vi "Pressure Control 1.vi"() -> ()   [LabVIEW 2013]
uses:
  <vilib>/DAQmx/write.llb/DAQmx Write.vi
  <vilib>/DAQmx/write.llb/DAQmx Write (Digital Bool 1Line 1Point).vi
  <vilib>/DAQmx/read.llb/DAQmx Read.vi
  <vilib>/DAQmx/read.llb/DAQmx Read (Analog DBL 1Chan 1Samp).vi
  <vilib>/Analysis/1siggen.llb/Ramp Pattern by Samples.vi
  support files/Pr Data Global.vi
  <vilib>/DAQmx/miscellaneous.llb/DAQmx Fill In Error Info.vi
  <vilib>/Analysis/NI_AALPro.lvlib
  <vilib>/Analysis/NI_AALBase.lvlib
panel:
  out "Delay Start":dbl format="%.2f"
  in  "Start Test":bool
  in  "quit":bool
  out "loops":bool
  out "Running?":bool
  in  "Tab":T1(tab)
  out "Vac":bool
  out "File Data:":T2 {"Min." format="%.2f"; "Ave." format="%.2f"; "Max." format="%.2f"}
  out "units 2":string
  out "units 1":string
  out "Relief":bool
  out "Pressure":bool
  out "Pr Data":sgl(graph)
  out "Ave. Pressure Input":sgl format="%.2f"
  out "Pressure Input":sgl format="%.2f"
  out "units 4":string
  out "units 3":string
  in  "Config Cluster":T3={"Pressure Setpoint"=20.0, "Deadband"=2.0, "Data Read Rate"=10.0, "Data Location"=1, "# Points to Ave."=2, "Data Storage"=FALSE, "Data Storage Rate"=10.0, "Data Path"=path "", "TR #"="", "Comp. ID"="", "Reset Buffer"=FALSE, "Reponse Time"=2.0} {"Reponse Time" min=0.0 max=10.0 format="%.1f"; "Data Storage Rate" format="%<%H:%M:%S>t"; "# Points to Ave." min=1 max=10000; "Data Location" min=1 max=10; "Data Read Rate" min=0.1 max=3600.0 format="%.1f"; "Deadband" format="%.2f"; "Pressure Setpoint" format="%.2f"}
  in  "IO Settings":T4={"Feedback Settings"={"Comm Resource"="Pr Module", "Device"="AI 120", "Item"="Channel 0"}, "Pressure Valve"={"Comm Resource"="Pr Module", "Device"="Relay", "Item"="Channel 0"}, "Relief Valve"={"Comm Resource"="Pr Module", "Device"="Relay", "Item"="Channel 0"}, "Vacuum Valve"={"Comm Resource"="Pr Module", "Device"="Relay", "Item"="Channel 0"}}
  in  "get amps":bool[](array[boolean])=[FALSE, FALSE, FALSE, FALSE, FALSE, FALSE]
  out "XY Graph":cluster{"Ramp Pattern":dbl[], dbl[]}[](graph)
  in  "Re-Calc":bool
  in  "Pr. Cal.":T5={"Model"="", "Gage #"="", "Cal Date"="", "Eng. Units"=[0.0, 0.0, 0.0, 0.0, 0.0, 0.0], "Amps"=[0.0, 0.0, 0.0, 0.0, 0.0, 0.0], "# Cal Points"=5, "Offset"=0.0, "Slope"=0.0, "Units"="kPa", "Master Gage #"=""} {"Slope" format="%.4f"; "Offset" format="%.4f"; "# Cal Points" min=2 max=6; "Amps" format="%.3f"; "Eng. Units" format="%.3f"}
  out "Data":sgl[][](array[numeric]) format="%.2f"
  # "(0.1-3600)"
  # "(0-10)"
  # "(1-10000)"
  # "(1-10)"
  # "(hh:mm:ss)"
  # "Pressure Input"
  # "(2-6)"
  # "min."
  # "max."
  # "ave."
  # "1"
  # "2"
  # "3"
  # "4"
  # "5"
  # "6"
  # "7"
  # "8"
  # "9"
  # "10"
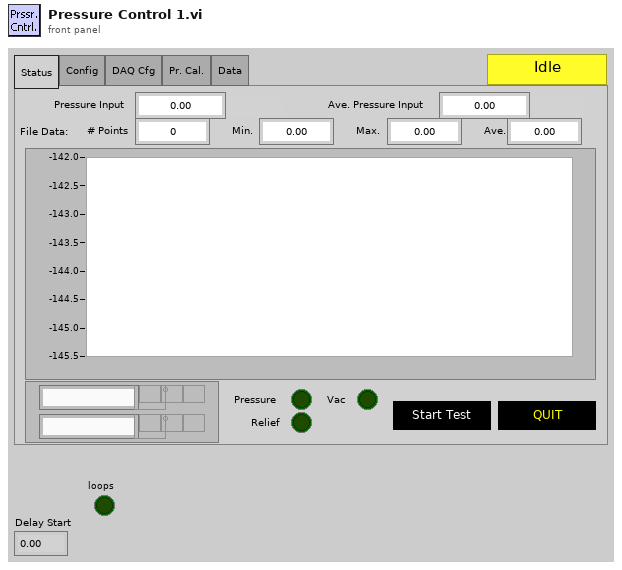
[diagram p1: front panel]
types:
  T1 = enum32{"Status", "Config", "DAQ Cfg", "Pr. Cal.", "Data"}
  T2 = cluster{"# Points":sgl, "Min.":sgl, "Max.":sgl, "Ave.":sgl}
  T3 = cluster{"Pressure Setpoint":dbl, "Deadband":dbl, "Data Read Rate":dbl, "Data Location":i32, "# Points to Ave.":i32, "Data Storage":bool, "Data Storage Rate":dbl, "Data Path":path, "TR #":string, "Comp. ID":string, "Reset Buffer":bool, "Reponse Time":dbl}
  T4 = cluster{"Feedback Settings":cluster{"Comm Resource":string, "Device":string, "Item":string}, "Pressure Valve":cluster{"Comm Resource":string, "Device":string, "Item":string}, "Relief Valve":cluster{"Comm Resource":string, "Device":string, "Item":string}, "Vacuum Valve":cluster{"Comm Resource":string, "Device":string, "Item":string}}
  T5 = cluster{"Model":string, "Gage #":string, "Cal Date":string, "Eng. Units":sgl[], "Amps":sgl[], "# Cal Points":u32, "Offset":sgl, "Slope":sgl, "Units":string, "Master Gage #":string}
  T6 = enum16{"Idle", "Adding Pr.", "Relieving Pr.", "Response Delay"}
  T7 = cluster{"IO Settings":cluster{"Feedback Settings":cluster{"Comm Resource":string, "Device":string, "Item":string}, "Pressure Valve":cluster{"Comm Resource":string, "Device":string, "Item":string}, "Relief Valve":cluster{"Comm Resource":string, "Device":string, "Item":string}, "Vacuum Valve":cluster{"Comm Resource":string, "Device":string, "Item":string}}, "Config Cluster":cluster{"Pressure Setpoint":dbl, "Deadband":dbl, "Data Read Rate":dbl, "Data Location":i32, "# Points to Ave.":i32, "Data Storage":bool, "Data Storage Rate":dbl, "Data Path":path, "TR #":string, "Comp. ID":string, "Reset Buffer":bool, "Reponse Time":dbl}, "Pr. Cal.":cluster{"Model":string, "Gage #":string, "Cal Date":string, "Eng. Units":sgl[], "Amps":sgl[], "# Cal Points":u32, "Offset":sgl, "Slope":sgl, "Units":string, "Master Gage #":string}}
  T8 = cluster{"# Pts, Min, Max, Ave.[0]":sgl, "# Pts, Min, Max, Ave.[1]":sgl, "# Pts, Min, Max, Ave.[2]":sgl, "# Pts, Min, Max, Ave.[3]":sgl}
  T9 = cluster{"Comm Resource":string, "Device":string, "Item":string}
  T10 = enum16{"open", "replace", "create", "open or create", "replace or create", "replace or create with confirmation"}
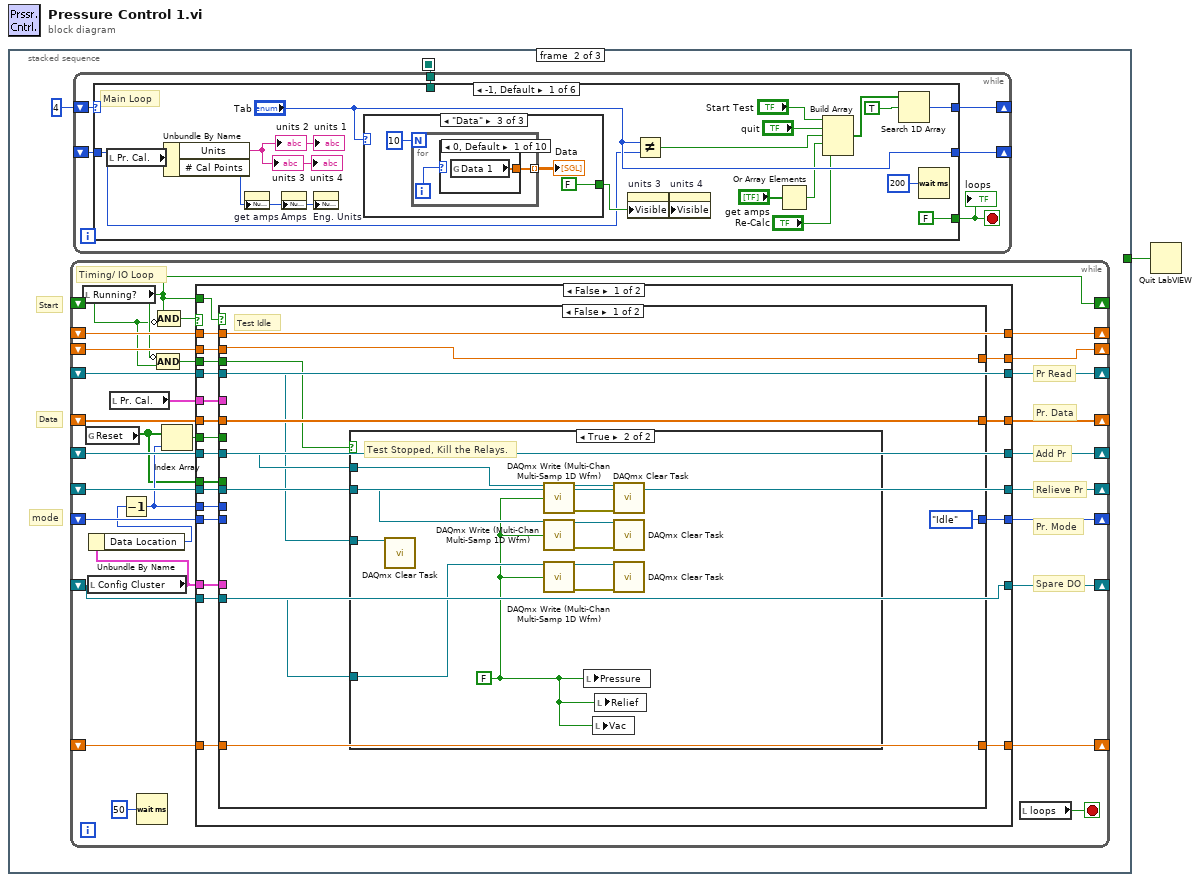
[diagram p0: block diagram]
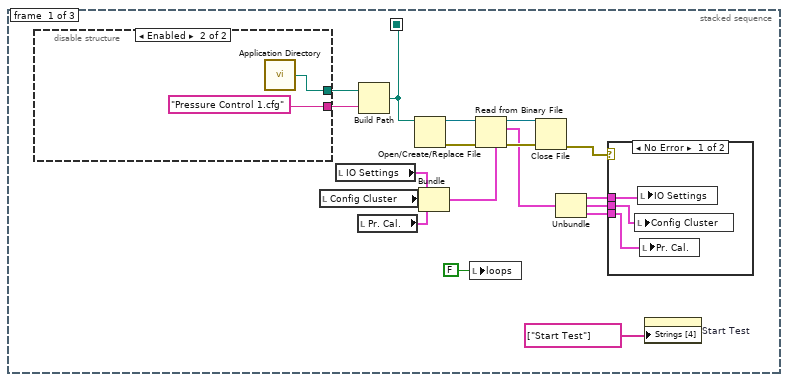
[diagram p2: hidden frame]
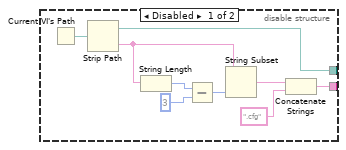
[diagram p3: hidden frame]
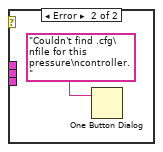
[diagram p4: hidden frame]
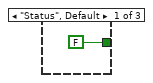
[diagram p5: hidden frame]
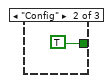
[diagram p6: hidden frame]
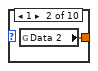
[diagram p7: hidden frame]
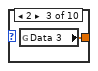
[diagram p8: hidden frame]
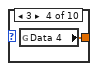
[diagram p9: hidden frame]
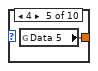
[diagram p10: hidden frame]
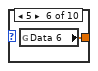
[diagram p11: hidden frame]
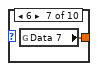
[diagram p12: hidden frame]
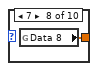
[diagram p13: hidden frame]
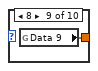
[diagram p14: hidden frame]
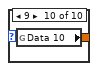
[diagram p15: hidden frame]
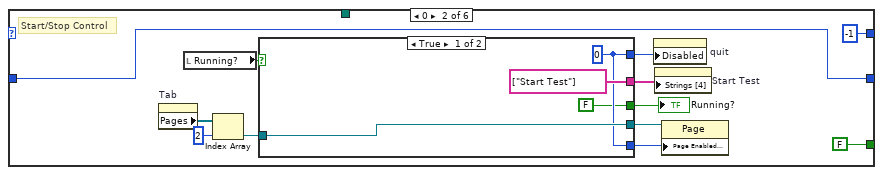
[diagram p16: hidden frame]
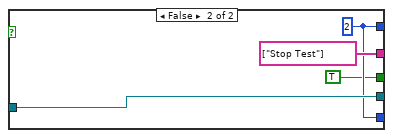
[diagram p17: hidden frame]
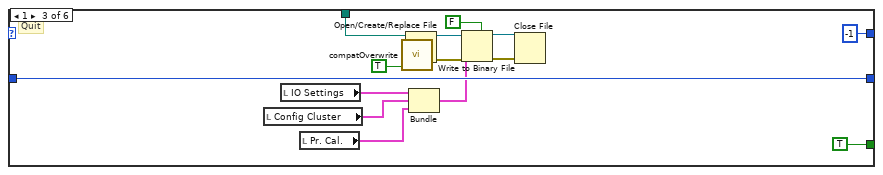
[diagram p18: hidden frame]
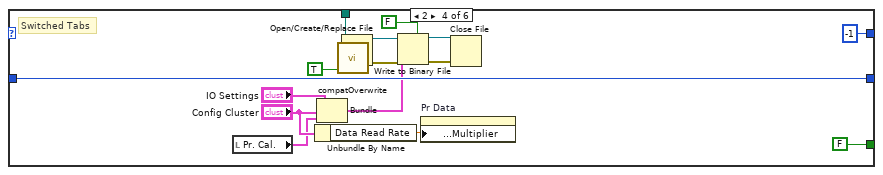
[diagram p19: hidden frame]
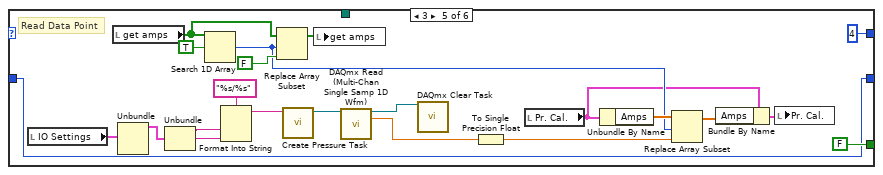
[diagram p20: hidden frame]
diagram:
  n1 = stacked-sequence {
    seq-local: [w17 _ _] -> [_ w36 _]
    tunnel: [_ _ TRUE ("quit? (T)")] -> w1
    frame #0 {
      n2 = disable-structure shown="Enabled" {
        disable-tunnel: [w21 "Pressure Control 1.cfg" ("Substring")] -> w19
        disable-tunnel: [w20 w30] -> w18
        frame Disabled {
          n3 = Current VI's Path() -> (path=w28:path)
          n4 = Strip Path(path=w28) -> (stripped path=w20:path, name=w27:string)
          n5 = String Length(string=w27) -> (length=w26:i32)
          n6 = Subtract(x=w26, y=3) -> (x-y=w22:i32)
          n7 = String Subset(string=w27, length (rest)=w22) -> (substring=w24:string)  [unwired: 1 in]
          n8 = Concatenate Strings(w24, ".cfg" ("Substring")) -> (w21:string)
        }
        frame Enabled {
          n9 = call <vilib>:"Application Directory.vi"() -> ("Application Directory"=w30:path)
        }
      }
      n10 = local read "Config Cluster"() -> (w16:T3)
      n11 = local read "IO Settings"() -> (w15:T4)
      n12 = local read "Pr. Cal."() -> (w4:T5)
      n13 = Build Path(base path=w18, name or relative path=w19) -> (appended path=w17:path)
      n14 = Open/Create/Replace File(file path (use dialog)=w17) -> (refnum out=w14:refnum<file>, error out=w13:errorcluster)  [unwired: 5 in, 1 out]
      n15 = Bundle("IO Settings"=w15, "Config Cluster"=w16, "Pr. Cal."=w4) -> (w12:T7)  [unwired: 1 in]
      n16 = local write "loops"(FALSE ("loops")) -> ()
      n17 = Read from Binary File(5:w12, 8:w13, 11:w14) -> (0:w11:errorcluster, 2:w8:T7, 3:w10:refnum<file>)  [unwired: 3 in, 1 out]
      n18 = Close File(refnum=w10, error in=w11) -> (error out=w9:errorcluster)  [unwired: 1 out]
      n19 = Unbundle(w8) -> ("IO Settings"=w7:T4, "Config Cluster"=w6:T3, "Pr. Cal."=w3:T5)
      n20 = case shown="No Error" w9 {
        tunnel: w7 -> [w33 _]
        tunnel: w6 -> [w32 _]
        tunnel: w3 -> [w31 _]
        frame No Error {
          n21 = local write "Config Cluster"(w32) -> ()
          n22 = local write "IO Settings"(w33) -> ()
          n23 = local write "Pr. Cal."(w31) -> ()
        }
        frame Error {
          n24 = One Button Dialog(message="Couldn't find .cfg\nfile for this pressure\ncontroller.") -> ()  [unwired: 1 in, 1 out]
        }
      }
      n25 = property on="Start Test" class="Bool"("Strings [4]"=string[] ["Start Test"]) -> ()  [unwired: 2 in, 2 out]
    }
    frame #1 {
      # "mode"
      # "Start"
      # "Data"
      n26 = while {
        shift-left: _ -> [w173]
        shift-right: [w174] -> _
        shift-left: _ -> [w184]
        shift-right: [w185] -> _
        shift-left: _ -> [w186]
        shift-right: [w189] -> _
        shift-left: _ -> [w187]
        shift-right: [w188] -> _
        shift-left: _ -> [w191]
        shift-right: [w194] -> _
        shift-left: _ -> [w192]
        shift-right: [w195] -> _
        shift-left: _ -> [w193]
        shift-right: [w196] -> _
        shift-left: _ -> [w190]
        shift-right: [w197] -> _
        shift-left: _ -> [w182]
        shift-right: [w183] -> _
        shift-right: [w172] -> _
        shift-left: _ -> [w171]
        stop <- w200 stop-if-true
        # "Spare DO"
        # "Pr. Mode"
        # "Pr. Data"
        # "Relieve Pr"
        # "Add Pr"
        # "Pr Read"
        # "Timing/ IO Loop"
        n27 = local read "Running?"() -> (w183:bool)
        n28 = global read "Pr Data Global.vi" "Reset"() -> (w175:bool[])
        n29 = local read "Config Cluster"() -> (w179:T3)
        n30 = Unbundle By Name(w179) -> ("Data Location"=w178:i32)
        n31 = local read "Pr. Cal."() -> (w180:T5)
        n32 = Decrement(x=w178) -> (x-1=w176:i32)
        n33 = Wait (ms)(milliseconds to wait=u32 50) -> ()  [unwired: 1 out]
        n34 = Compound Arithmetic op=AND(invert w183, w182) -> (w181:bool)
        n35 = Compound Arithmetic op=AND(w183, invert w182) -> (w199:bool)
        n36 = Index Array(array=w175, index=w176) -> (element=w177:bool)
        n37 = case shown="False" w199 {
          tunnel: [w220 w431] -> w197
          tunnel: [w218 w427] -> w196
          tunnel: [w217 w426] -> w195
          tunnel: [w216 w430] -> w194
          tunnel: w193 -> [w218 _]
          tunnel: w192 -> [w217 _]
          tunnel: w191 -> [w216 _]
          tunnel: w190 -> [w220 _]
          tunnel: w183 -> [w219 _]
          tunnel: w179 -> [w215 _]
          tunnel: [w211 0.0] -> w189
          tunnel: [w213 sgl[] []] -> w188
          tunnel: w187 -> [w214 _]
          tunnel: w186 -> [w212 _]
          tunnel: [w209 T6."Idle"] -> w185
          tunnel: w184 -> [w210 _]
          tunnel: w181 -> [w208 _]
          tunnel: w180 -> [w207 _]
          tunnel: w177 -> [w206 _]
          tunnel: w176 -> [w205 _]
          tunnel: w175 -> [w204 _]
          tunnel: [w203 0.0] -> w174
          tunnel: w173 -> [w202 _]
          tunnel: [w201 w398] -> w172
          tunnel: w171 -> [w201 _]
          frame False {
            n38 = case shown="False" w219 {
              tunnel: w220 -> [_ w281]
              tunnel: w218 -> [w222 w279]
              tunnel: w217 -> [w225 w268]
              tunnel: w216 -> [w224 w263]
              tunnel: w215 -> [_ w253]
              tunnel: w214 -> [w229 w249]
              tunnel: [w229 w273] -> w213
              tunnel: w212 -> [w228 w277]
              tunnel: [w228 w276] -> w211
              tunnel: [T6."Idle" w269] -> w209
              tunnel: w210 -> [_ w272]
              tunnel: w208 -> [w226 _]
              tunnel: w207 -> [_ w267]
              tunnel: w206 -> [_ w251]
              tunnel: w205 -> [_ w262]
              tunnel: w204 -> [_ w261]
              tunnel: [w223 w258] -> w203
              tunnel: w202 -> [w223 w257]
              tunnel: w201 -> [w221 w241]
              frame False {
                # "Test Idle"
                n39 = case shown="True" w226 {
                  tunnel: w225 -> [_ w240]
                  tunnel: w224 -> [_ w239]
                  tunnel: w222 -> [_ w234]
                  tunnel: w221 -> [_ w231]
                  frame False {
                  }
                  frame True {
                    w230 = FALSE ("value")
                    # "Test Stopped, Kill the Relays."
                    n40 = call <vilib>:"DAQmx Clear Task.vi"("task in"=w234) -> ()  [unwired: 14 in, 1 out]
                    n41 = call-poly "DAQmx Write (Multi-Chan Multi-Samp 1D Wfm).vi"("task/channels in"=w240, "data"=w230) -> ("task out"=w238:refnum<k21>, "error out"=w237:errorcluster)  [unwired: 11 in, 1 out]
                    n42 = call-poly "DAQmx Write (Multi-Chan Multi-Samp 1D Wfm).vi"("task/channels in"=w239, "data"=w230) -> ("task out"=w236:refnum<k21>, "error out"=w235:errorcluster)  [unwired: 11 in, 1 out]
                    n43 = call-poly "DAQmx Write (Multi-Chan Multi-Samp 1D Wfm).vi"("task/channels in"=w231, "data"=w230) -> ("task out"=w232:refnum<k21>, "error out"=w233:errorcluster)  [unwired: 11 in, 1 out]
                    n44 = local write "Pressure"(w230) -> ()
                    n45 = local write "Vac"(w230) -> ()
                    n46 = local write "Relief"(w230) -> ()
                    n47 = call <vilib>:"DAQmx Clear Task.vi"("task in"=w238, "error in"=w237) -> ()  [unwired: 13 in, 1 out]
                    n48 = call <vilib>:"DAQmx Clear Task.vi"("task in"=w236, "error in"=w235) -> ()  [unwired: 13 in, 1 out]
                    n49 = call <vilib>:"DAQmx Clear Task.vi"("task in"=w232, "error in"=w233) -> ()  [unwired: 13 in, 1 out]
                  }
                }
              }
              frame True {
                # "Test running"
                n50 = Unbundle By Name(w253) -> ("Reponse Time"=w245:dbl, "Data Read Rate"=w278:dbl, "# Points to Ave."=w274:i32, "Data Location"=w254:i32, "Pressure Setpoint"=w243:dbl, "Deadband"=w270:dbl, "Data Storage"=w256:bool, "Data Storage Rate"=w259:dbl, "Reset Buffer"=w248:bool)
                n51 = case shown="True" w251 {
                  tunnel: w262 -> [_ w288]
                  tunnel: w261 -> [_ w287]
                  frame False {
                  }
                  frame True {
                    n52 = Replace Array Subset(array=w287, new element=FALSE ("New Element/Subarray"), index=w288) -> (w286:bool[])
                    n53 = global write "Pr Data Global.vi" "Reset"(w286) -> ()
                  }
                }
                n54 = Get Date/Time In Seconds() -> (seconds since 1Jan1904=w244:timestamp)
                n55 = Unbundle By Name(w267) -> ("Slope"=w266:sgl, "Offset"=w265:sgl)
                n56 = To Double Precision Float(number=w244) -> (double precision float=w280:dbl)
                n57 = Subtract(x=w281, y=w280) -> (x-y=w260:dbl)
                n58 = Quotient & Remainder(x=w260, y=w278) -> (floor(x/y)=w276:dbl)  [unwired: 1 out]
                n59 = Quotient & Remainder(x=w260, y=w259) -> (floor(x/y)=w258:dbl)  [unwired: 1 out]
                n60 = Greater Or Equal To 0?(x=w243) -> (x >= 0?=w242:bool)
                n61 = Not Equal?(x=w276, y=w277) -> (x != y?=w275:bool)
                n62 = Not Equal?(x=w258, y=w257) -> (x != y?=w247:bool)
                n63 = And(x=w247, y=w248) -> (x .and. y?=w246:bool)
                n64 = Or(x=w251, y=w246) -> (x .or. y?=w252:bool)
                n65 = Select(t=sgl[] [], s=w252, f=w249) -> (s? t:f=w250:sgl[])
                n66 = case shown="True" w275 {
                  tunnel: w279 -> [_ w372]
                  tunnel: w250 -> [w369 w387]
                  tunnel: w274 -> [_ w386]
                  tunnel: [w369 w375] -> w273
                  tunnel: w254 -> [_ w385]
                  tunnel: [w368 w370] -> w271
                  tunnel: w266 -> [_ w383]
                  tunnel: w265 -> [_ w380]
                  frame False {
                    # "Not time to take data point"
                    n67 = local read "Ave. Pressure Input"() -> (w368:sgl)
                  }
                  frame True {
                    n68 = call-poly "DAQmx Read (Multi-Chan Single Samp 1D Wfm).vi"("task/channels in"=w372) -> ("data"=w371:dbl)  [unwired: 12 in, 2 out]
                    n69 = To Single Precision Float(number=w371) -> (single precision float=w379:sgl)
                    n70 = Multiply(x=w383, y=w379) -> (x*y=w382:sgl)
                    n71 = Add(x=w382, y=w380) -> (x+y=w381:sgl)
                    "Pressure Input" <- w381
                    "Pr Data" <- w381
                    n72 = Build Array (concatenate)(w381, w387) -> (w375:sgl[])
                    n73 = Array Subset(array=w375, length=w386) -> (w378:sgl[])  [unwired: 1 in]
                    n74 = call "Min Max and Ave.vi"("Data In"=w378) -> ("Ave. Pressure Input"=w370:sgl)  [unwired: 1 in, 1 out]
                    "Ave. Pressure Input" <- w370
                    n75 = call "Min Max and Ave.vi"("Data In"=w375) -> ("# Pts, Min, Max, Ave."=w373:sgl[])  [unwired: 1 in, 1 out]
                    n76 = Array To Cluster(array=w373) -> (cluster=→"File Data:":T8)
                    n77 = Array Subset(array=w373, index=1 ("Array Index")) -> (w376:sgl[])  [unwired: 1 in]
                    n78 = Decrement(x=w385) -> (x-1=w384:i32)
                    n79 = case shown="0, Default" w384 {
                      tunnel: w376 -> [w388 w389 w390 w391 w392 w393 w394 w395 w396 w397]
                      frame 0, Default {
                        n80 = global write "Pr Data Global.vi" "Data 1"(w388) -> ()
                      }
                      frame 1 {
                        n81 = global write "Pr Data Global.vi" "Data 2"(w389) -> ()
                      }
                      frame 2 {
                        n82 = global write "Pr Data Global.vi" "Data 3"(w390) -> ()
                      }
                      frame 3 {
                        n83 = global write "Pr Data Global.vi" "Data 4"(w391) -> ()
                      }
                      frame 4 {
                        n84 = global write "Pr Data Global.vi" "Data 5"(w392) -> ()
                      }
                      frame 5 {
                        n85 = global write "Pr Data Global.vi" "Data 6"(w393) -> ()
                      }
                      frame 6 {
                        n86 = global write "Pr Data Global.vi" "Data 7"(w394) -> ()
                      }
                      frame 7 {
                        n87 = global write "Pr Data Global.vi" "Data 8"(w395) -> ()
                      }
                      frame 8 {
                        n88 = global write "Pr Data Global.vi" "Data 9"(w396) -> ()
                      }
                      frame 9 {
                        n89 = global write "Pr Data Global.vi" "Data 10"(w397) -> ()
                      }
                    }
                  }
                }
                n90 = case shown="\"Idle\", Default" w272 {
                  tunnel: w271 -> [w291 w329 w347 _]
                  tunnel: w243 -> [w300 w328 w346 _]
                  tunnel: w270 -> [w299 _ _ _]
                  tunnel: [w295 w326 w344 w360] -> w269
                  tunnel: w268 -> [w294 w325 _ _]
                  tunnel: w263 -> [w293 w323 w343 _]
                  tunnel: w245 -> [_ _ _ w364]
                  tunnel: w242 -> [w290 w324 w342 _]
                  tunnel: w241 -> [w289 _ w341 _]
                  frame "Idle", Default {
                    # "adjust PR?"
                    n91 = Add(x=w300, y=w299) -> (x+y=w298:dbl)
                    n92 = Subtract(x=w300, y=w299) -> (x-y=w292:dbl)
                    n93 = Greater?(x=w291, y=w298) -> (0:w297:bool)
                    n94 = Less?(x=w291, y=w292) -> (x < y?=w296:bool)
                    n95 = case shown="False" w297 {
                      tunnel: w296 -> [w305 _]
                      tunnel: [w304 T6."Relieving Pr."] -> w295
                      tunnel: w294 -> [w303 _]
                      tunnel: w293 -> [w301 w316]
                      tunnel: w290 -> [w302 w317]
                      tunnel: w289 -> [_ w315]
                      frame False {
                        n96 = case shown="True" w305 {
                          tunnel: [T6."Idle" T6."Adding Pr."] -> w304
                          tunnel: w303 -> [_ w309]
                          tunnel: w302 -> [_ w308]
                          tunnel: w301 -> [_ w307]
                          frame False {
                            # "Pressure Still OK"
                          }
                          frame True {
                            # "Start Adding Pressure"
                            n97 = case shown="False" w308 {
                              tunnel: w309 -> [w312 _]
                              tunnel: w307 -> [_ w314]
                              frame True {
                                w311 = TRUE ("value")
                                # "Use pressure valve since \nsetpoint is positive."
                                n98 = call-poly "DAQmx Write (Multi-Chan Multi-Samp 1D Wfm).vi"("task/channels in"=w312, "data"=w311) -> ()  [unwired: 11 in, 3 out]
                                "Pressure" <- w311
                              }
                              frame False {
                                w313 = TRUE ("value")
                                # "Use relief valve since \nsetpoint is negative."
                                n99 = call-poly "DAQmx Write (Multi-Chan Multi-Samp 1D Wfm).vi"("task/channels in"=w314, "data"=w313) -> ()  [unwired: 11 in, 3 out]
                                n100 = local write "Relief"(w313) -> ()
                              }
                            }
                          }
                        }
                      }
                      frame True {
                        # "Start Relieving Pressure"
                        n101 = case shown="True" w317 {
                          tunnel: w316 -> [w319 _]
                          tunnel: w315 -> [_ w321]
                          frame True {
                            w320 = TRUE ("value")
                            # "Use relief valve since setpoint\nis positive"
                            n102 = call-poly "DAQmx Write (Multi-Chan Multi-Samp 1D Wfm).vi"("task/channels in"=w319, "data"=w320) -> ()  [unwired: 11 in, 3 out]
                            "Relief" <- w320
                          }
                          frame False {
                            w322 = TRUE ("value")
                            # "Use vac valve since setpoint\nis negative."
                            n103 = call-poly "DAQmx Write (Multi-Chan Multi-Samp 1D Wfm).vi"("task/channels in"=w321, "data"=w322) -> ()  [unwired: 11 in, 3 out]
                            "Vac" <- w322
                          }
                        }
                      }
                    }
                  }
                  frame "Adding Pr." {
                    # "Stop Adding when pr. hits setpoint"
                    n104 = Greater Or Equal?(x=w329, y=w328) -> (x >= y?=w327:bool)
                    n105 = case shown="True" w327 {
                      tunnel: [T6."Adding Pr." T6."Response Delay"] -> w326
                      tunnel: w325 -> [_ w332]
                      tunnel: w324 -> [_ w333]
                      tunnel: w323 -> [_ w331]
                      frame False {
                        # "Still Adding PR."
                      }
                      frame True {
                        # "Pressure hit Setpoint, close Pr. valve"
                        n106 = case shown="True" w333 {
                          tunnel: w332 -> [w338 _]
                          tunnel: w331 -> [_ w339]
                          frame True {
                            w337 = FALSE ("value")
                            # "Use pressure valve since \nsetpoint is positive."
                            n107 = call-poly "DAQmx Write (Multi-Chan Multi-Samp 1D Wfm).vi"("task/channels in"=w338, "data"=w337) -> ()  [unwired: 11 in, 3 out]
                            n108 = local write "Pressure"(w337) -> ()
                          }
                          frame False {
                            w340 = FALSE ("value")
                            # "Use relief valve since \nsetpoint is negative."
                            n109 = call-poly "DAQmx Write (Multi-Chan Multi-Samp 1D Wfm).vi"("task/channels in"=w339, "data"=w340) -> ()  [unwired: 11 in, 3 out]
                            n110 = local write "Relief"(w340) -> ()
                          }
                        }
                        n111 = Get Date/Time In Seconds() -> (seconds since 1Jan1904=w334:timestamp)
                        n112 = To Double Precision Float(number=w334) -> (double precision float=→"Delay Start":dbl)
                      }
                    }
                  }
                  frame "Relieving Pr." {
                    # "Stop relieving when pr. hits setpoint"
                    n113 = Less Or Equal?(x=w347, y=w346) -> (x <= y?=w345:bool)
                    n114 = case shown="True" w345 {
                      tunnel: [T6."Relieving Pr." T6."Response Delay"] -> w344
                      tunnel: w343 -> [_ w351]
                      tunnel: w342 -> [_ w350]
                      tunnel: w341 -> [_ w349]
                      frame False {
                        # "Still relieving PR."
                      }
                      frame True {
                        # "Pressure hit Setpoint, close relief valve"
                        n115 = case shown="False" w350 {
                          tunnel: w351 -> [w356 _]
                          tunnel: w349 -> [_ w357]
                          frame True {
                            w355 = FALSE ("value")
                            # "Use relief valve since \nsetpoint is positive."
                            n116 = local write "Relief"(w355) -> ()
                            n117 = call-poly "DAQmx Write (Multi-Chan Multi-Samp 1D Wfm).vi"("task/channels in"=w356, "data"=w355) -> ()  [unwired: 11 in, 3 out]
                          }
                          frame False {
                            w358 = FALSE ("value")
                            # "Use vac valve since \nsetpoint is negative."
                            n118 = call-poly "DAQmx Write (Multi-Chan Multi-Samp 1D Wfm).vi"("task/channels in"=w357, "data"=w358) -> ()  [unwired: 11 in, 3 out]
                            n119 = local write "Vac"(w358) -> ()
                          }
                        }
                        n120 = Get Date/Time In Seconds() -> (seconds since 1Jan1904=w352:timestamp)
                        n121 = To Double Precision Float(number=w352) -> (double precision float=w353:dbl)
                        n122 = local write "Delay Start"(w353) -> ()
                      }
                    }
                  }
                  frame "Response Delay" {
                    # "Wait for system to stabilize before adding or relieving anymore pressure"
                    n123 = local read "Delay Start"() -> (w366:dbl)
                    n124 = Get Date/Time In Seconds() -> (seconds since 1Jan1904=w359:timestamp)
                    n125 = To Double Precision Float(number=w359) -> (double precision float=w367:dbl)
                    n126 = Subtract(x=w367, y=w366) -> (x-y=w365:dbl)
                    n127 = Greater Or Equal?(x=w365, y=w364) -> (x >= y?=w363:bool)
                    n128 = Select(t=T6."Idle", s=w363, f=T6."Response Delay") -> (s? t:f=w360:T6)
                  }
                }
                n129 = And(x=w256, y=w247) -> (x .and. y?=w255:bool)
                n130 = case shown="True" w255 {
                  tunnel: w253 -> [_ w284]
                  tunnel: w249 -> [_ w283]
                  frame False {
                  }
                  frame True {
                    n131 = local read "Pr. Cal."() -> (w282:T5)
                    n132 = call "Save Data.vi"("Data Buffer"=w283, "Config Cluster"=w284, "Pr. Cal."=w282) -> ()  [unwired: 3 in]
                  }
                }
              }
            }
          }
          frame True {
            (unwired) "cDAQ1Mod1/ai0" ("physical channel")
            (unwired) "cDAQ1Mod2/port0/line0" ("Line")
            # "Reset Ref#s, Timer"
            n133 = local read "IO Settings"() -> (w420:T4)
            n134 = Unbundle(w420) -> ("Feedback Settings"=w422:T9, "Pressure Valve"=w421:T9, "Relief Valve"=w407:T9, "Vacuum Valve"=w399:T9)
            n135 = Unbundle(w422) -> ("Comm Resource"=w419:string, "Device"=w418:string)  [unwired: 1 out]
            n136 = Unbundle(w421) -> ("Comm Resource"=w414:string, "Device"=w413:string, "Item"=w412:string)
            n137 = Unbundle(w407) -> ("Comm Resource"=w409:string, "Device"=w410:string, "Item"=w411:string)
            n138 = Unbundle(w399) -> ("Comm Resource"=w403:string, "Device"=w402:string, "Item"=w401:string)
            n139 = Format Into String(format string="%s/%s", w419, w418) -> (resulting string=w416:string)  [unwired: 2 in, 1 out]
            n140 = Format Into String(format string="%s/%s/%s", w414, w413, w412) -> (resulting string=w406:string)  [unwired: 2 in, 1 out]
            n141 = Format Into String(format string="%s/%s/%s", w409, w410, w411) -> (resulting string=w405:string)  [unwired: 2 in, 1 out]
            n142 = Format Into String(format string="%s/%s/%s", w403, w402, w401) -> (resulting string=w400:string)  [unwired: 2 in, 1 out]
            n143 = call "Create Pressure Task.vi"("physical channel"=w416) -> ("task out"=w427:refnum<k21>)  [unwired: 9 in, 1 out]
            n144 = call "Create DO Task.vi"("Line"=w406) -> ("task out"=w426:refnum<k21>)  [unwired: 9 in, 1 out]
            n145 = call "Create DO Task.vi"("Line"=w405) -> ("task out"=w430:refnum<k21>)  [unwired: 9 in, 1 out]
            n146 = call "Create DO Task.vi"("Line"=w400) -> ("task out"=w398:refnum<k21>)  [unwired: 9 in, 1 out]
            n147 = Get Date/Time In Seconds() -> (seconds since 1Jan1904=w423:timestamp)
            n148 = To Double Precision Float(number=w423) -> (double precision float=w431:dbl)
          }
        }
        n149 = local read "loops"() -> (w200:bool)
      }
      n150 = while {
        tunnel: w36 -> [w37]
        shift-left: _ -> [w40]
        shift-right: [w39] -> _
        shift-left: 4 ("index of element") -> [w41]
        shift-right: [w42] -> _
        stop <- w38 stop-if-true
        n151 = case shown="-1, Default" w41 {
          tunnel: [w56 -1 ("index of element") -1 ("index of element") -1 ("index of element") 4 ("index of element") -1 ("index of element")] -> w42
          tunnel: w40 -> [w45 w79 w110 w126 w146 w168]
          tunnel: ["Tab" w79 w110 w126 w146 w168] -> w39
          tunnel: [FALSE FALSE TRUE ("T button?") FALSE ("T button?") FALSE ("T button?") FALSE ("T button?")] -> w38
          tunnel: w37 -> [_ _ w100 w123 _ _]
          frame -1, Default {
            # "Main Loop"
            n152 = local read "Pr. Cal."() -> (w47:T5)
            n153 = Unbundle By Name(w47) -> ("Units"=→"units 1" →"units 2" →"units 4" →"units 3":string, "# Cal Points"=w44:u32)
            n154 = property on="get amps" class="Arr"("Number of Rows"=w44) -> ()  [unwired: 2 in, 2 out]
            n155 = property on="Amps" class="Arr (strict)"("Number of Rows"=w44) -> ()  [unwired: 2 in, 2 out]
            n156 = property on="Eng. Units" class="Arr (strict)"("Number of Rows"=w44) -> ()  [unwired: 2 in, 2 out]
            n157 = case shown="\"Data\"" "Tab" {
              tunnel: [FALSE ("Visible") TRUE ("Visible") FALSE ("Visible")] -> w50
              frame "Status", Default {
              }
              frame "Config" {
              }
              frame "Data" {
                n158 = for {
                  N: 10 -> [_]
                  tunnel: [w65] -> w63 mode=indexing
                  i -> [w66]
                  n159 = case shown="0, Default" w66 {
                    tunnel: [w67 w68 w69 w70 w71 w72 w73 w74 w75 w76] -> w65
                    frame 0, Default {
                      n160 = global read "Pr Data Global.vi" "Data 1"() -> (w67:sgl[])
                    }
                    frame 1 {
                      n161 = global read "Pr Data Global.vi" "Data 2"() -> (w68:sgl[])
                    }
                    frame 2 {
                      n162 = global read "Pr Data Global.vi" "Data 3"() -> (w69:sgl[])
                    }
                    frame 3 {
                      n163 = global read "Pr Data Global.vi" "Data 4"() -> (w70:sgl[])
                    }
                    frame 4 {
                      n164 = global read "Pr Data Global.vi" "Data 5"() -> (w71:sgl[])
                    }
                    frame 5 {
                      n165 = global read "Pr Data Global.vi" "Data 6"() -> (w72:sgl[])
                    }
                    frame 6 {
                      n166 = global read "Pr Data Global.vi" "Data 7"() -> (w73:sgl[])
                    }
                    frame 7 {
                      n167 = global read "Pr Data Global.vi" "Data 8"() -> (w74:sgl[])
                    }
                    frame 8 {
                      n168 = global read "Pr Data Global.vi" "Data 9"() -> (w75:sgl[])
                    }
                    frame 9 {
                      n169 = global read "Pr Data Global.vi" "Data 10"() -> (w76:sgl[])
                    }
                  }
                }
                "Data" <- w63
              }
            }
            n170 = property on="units 3" class="Str"("Visible"=w50) -> ()  [unwired: 2 in, 2 out]
            n171 = Not Equal?(x="Tab", y=w45) -> (x != y?=w53:bool)
            n172 = property on="units 4" class="Str"("Visible"=w50) -> ()  [unwired: 2 in, 2 out]
            n173 = Or Array Elements(Boolean array="get amps") -> (logical OR=w48:bool)
            n174 = Build Array("Start Test", "quit", w53, w48, "Re-Calc") -> (w59:bool[])
            n175 = Search 1D Array(1D array=w59, element=TRUE) -> (index of element=w56:i32)  [unwired: 1 in]
            n176 = Wait (ms)(milliseconds to wait=u32 200) -> ()  [unwired: 1 out]
          }
          frame 0 {
            # "Start/Stop Control"
            n177 = property on="Tab" class="TabCtl (strict)"() -> ("Pages"=w85:refnum<vi>[])  [unwired: 2 in, 2 out]
            n178 = local read "Running?"() -> (w88:bool)
            n179 = Index Array(array=w85, index=2 ("Index")) -> (element=w83:refnum<vi>)
            n180 = case shown="True" w88 {
              tunnel: [string[] ["Start Test"] ("Strings [4]") string[] ["Stop Test"] ("Strings [4]")] -> w87
              tunnel: [w90 w94] -> w86
              tunnel: [w91 w95] -> w82
              tunnel: w83 -> [w91 w95]
              tunnel: [w90 w94] -> w81
              tunnel: [FALSE ("Running?") TRUE ("Running?")] -> w77
              frame True {
                w90 = u8 0 ("Disabled")
              }
              frame False {
                w94 = u8 2 ("Disabled")
              }
            }
            "Running?" <- w77
            n181 = property on="quit" class="Bool"("Disabled"=w86) -> ()  [unwired: 2 in, 2 out]
            n182 = property on="Start Test" class="Bool"("Strings [4]"=w87) -> ()  [unwired: 2 in, 2 out]
            n183 = property class="Page"(reference=w82, "Page Enabled State"=w81) -> ()  [unwired: 1 in, 2 out]
          }
          frame 1 {
            # "Quit"
            n184 = local read "Config Cluster"() -> (w108:T3)
            n185 = local read "IO Settings"() -> (w107:T4)
            n186 = local read "Pr. Cal."() -> (w99:T5)
            n187 = call <vilib>:"compatOverwrite.vi"("overwrite (F)"=TRUE) -> ("overwrite?"=w97:T10)
            n188 = Open/Create/Replace File(file path (use dialog)=w100, operation (0:open)=w97) -> (refnum out=w105:refnum<file>, error out=w104:errorcluster)  [unwired: 4 in, 1 out]
            n189 = Bundle("IO Settings"=w107, "Config Cluster"=w108, "Pr. Cal."=w99) -> (w106:T7)  [unwired: 1 in]
            n190 = Write to Binary File(file (use dialog)=w105, data=w106, error in=w104, 5:FALSE ("prepend array or string size? (T)")) -> (refnum out=w103:refnum<file>, error out=w102:errorcluster)  [unwired: 2 in, 1 out]
            n191 = Close File(refnum=w103, error in=w102) -> ()  [unwired: 2 out]
          }
          frame 2 {
            # "Switched Tabs"
            n192 = local read "Pr. Cal."() -> (w114:T5)
            n193 = Unbundle By Name("Config Cluster") -> ("Data Read Rate"=w115:dbl)
            n194 = Bundle("IO Settings"="IO Settings", "Config Cluster"="Config Cluster", "Pr. Cal."=w114) -> (w120:T7)  [unwired: 1 in]
            n195 = call <vilib>:"compatOverwrite.vi"("overwrite (F)"=TRUE) -> ("overwrite?"=w112:T10)
            n196 = Open/Create/Replace File(file path (use dialog)=w123, operation (0:open)=w112) -> (refnum out=w122:refnum<file>, error out=w121:errorcluster)  [unwired: 4 in, 1 out]
            n197 = Write to Binary File(file (use dialog)=w122, data=w120, error in=w121, 5:FALSE ("prepend array or string size? (T)")) -> (refnum out=w119:refnum<file>, error out=w118:errorcluster)  [unwired: 2 in, 1 out]
            n198 = property on="Pr Data" class="WFChart (strict)"("X Scale.Offset and Multiplier:Multiplier"=w115) -> ()  [unwired: 2 in, 2 out]
            n199 = Close File(refnum=w119, error in=w118) -> ()  [unwired: 2 out]
          }
          frame 3 {
            # "Read Data Point"
            n200 = local read "IO Settings"() -> (w147:T4)
            n201 = local read "get amps"() -> (w144:bool[])
            n202 = Unbundle(w147) -> ("Feedback Settings"=w135:T9)  [unwired: 3 out]
            n203 = Unbundle(w135) -> ("Comm Resource"=w133:string, "Device"=w132:string)  [unwired: 1 out]
            n204 = Search 1D Array(1D array=w144, element=TRUE) -> (index of element=w140:i32)  [unwired: 1 in]
            n205 = Format Into String(format string="%s/%s", w133, w132) -> (resulting string=w131:string)  [unwired: 2 in, 1 out]
            n206 = Replace Array Subset(array=w144, new element=FALSE ("New Element/Subarray"), index=w140) -> (w143:bool[])
            n207 = call "Create Pressure Task.vi"("physical channel"=w131) -> ("task out"=w130:refnum<k21>)  [unwired: 9 in, 1 out]
            n208 = local write "get amps"(w143) -> ()
            n209 = call-poly "DAQmx Read (Multi-Chan Single Samp 1D Wfm).vi"("task/channels in"=w130) -> ("task out"=w128:refnum<k21>, "data"=w129:dbl)  [unwired: 12 in, 1 out]
            n210 = call <vilib>:"DAQmx Clear Task.vi"("task in"=w128) -> ()  [unwired: 14 in, 1 out]
            n211 = To Single Precision Float(number=w129) -> (single precision float=w139:sgl)
            n212 = local read "Pr. Cal."() -> (w138:T5)
            n213 = Unbundle By Name(w138) -> ("Amps"=w141:sgl[])
            n214 = Replace Array Subset(array=w141, new element=w139, index=w140) -> (w137:sgl[])
            n215 = Bundle By Name(cluster=w138, "Amps"=w137) -> (w136:T5)
            n216 = local write "Pr. Cal."(w136) -> ()
          }
          frame 4 {
            # "Re-Draw Cal Graph"
            n217 = Unbundle By Name("Pr. Cal.") -> ("Amps"=w162:sgl[], "Eng. Units"=w163:sgl[], "# Cal Points"=w165:u32)
            n218 = Array Subset(array=w162, length=w165) -> (w160:sgl[])  [unwired: 1 in]
            n219 = Array Subset(array=w163, length=w165) -> (w161:sgl[])  [unwired: 1 in]
            n220 = Bundle(w160, w161) -> (w158:cluster{sgl[], sgl[]})  [unwired: 1 in]
            n221 = call <vilib>:"Linear Fit Coefficients.vi"("Y"=w161, "X"=w160) -> ("slope"=w151:dbl, "intercept"=w150:dbl)  [unwired: 11 in, 1 out]
            n222 = call-poly <vilib>:"Ramp Pattern.vi"("start"=0.02, "end"=0.004) -> ("Ramp Pattern"=w155:dbl[])  [unwired: 8 in, 1 out]
            n223 = Multiply(x=w155, y=w151) -> (x*y=w154:dbl[])
            n224 = Add(x=w154, y=w150) -> (x+y=w156:dbl[])
            n225 = Bundle("Ramp Pattern"=w155, w156) -> (w157:cluster{"Ramp Pattern":dbl[], dbl[]})  [unwired: 1 in]
            n226 = Build Array(w157, w158) -> (→"XY Graph":cluster{"Ramp Pattern":dbl[], dbl[]}[])
            n227 = local read "Pr. Cal."() -> (w167:T5)
            n228 = Bundle By Name(cluster=w167, "Slope"=w151, "Offset"=w150) -> (w166:T5)
            n229 = local write "Pr. Cal."(w166) -> ()
          }
        }
        "loops" <- w38
      }
    }
    frame #2 {
      n230 = Current VI's Path() -> (path=w433:path)
      n231 = Open VI Reference(vi path=w433) -> (vi reference=w434:refnum<vi>)  [unwired: 5 in, 1 out]
      n232 = property class="VI"(reference=w434, "Front Panel Window:Open"=FALSE) -> ()  [unwired: 1 in, 2 out]
    }
  }
  n233 = Quit LabVIEW(quit? (T)=w1) -> ()
